vi "CRYTree Structure Update.vi"(8 "Is Refresh?":bool, 9 "Option":string, 10 "Add Items":T1(array[cluster]), 11 "StepsRef in":refnum<vi>) -> (0 "error out":errorcluster, 3 "StepsRefOut":refnum<vi>)   [LabVIEW 2013]
uses:
  <vilib>/Utility/miscctls.llb/LVNodeAndColumnTypeDef.ctl
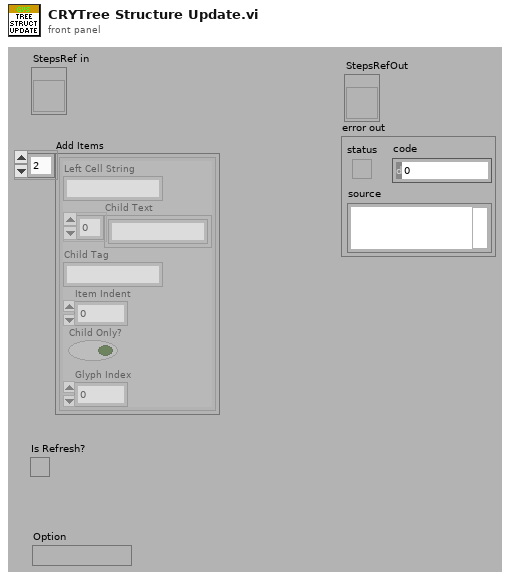
[diagram p1: front panel]
types:
  T1 = cluster{"Left Cell String":string, "Child Text":string[], "Child Tag":string, "Item Indent":i32, "Child Only?":bool, "Glyph Index":i32}[]
  T2 = typedef "LVNodeAndColumnTypeDef.ctl" = cluster{"Node":string, "Column":i32}
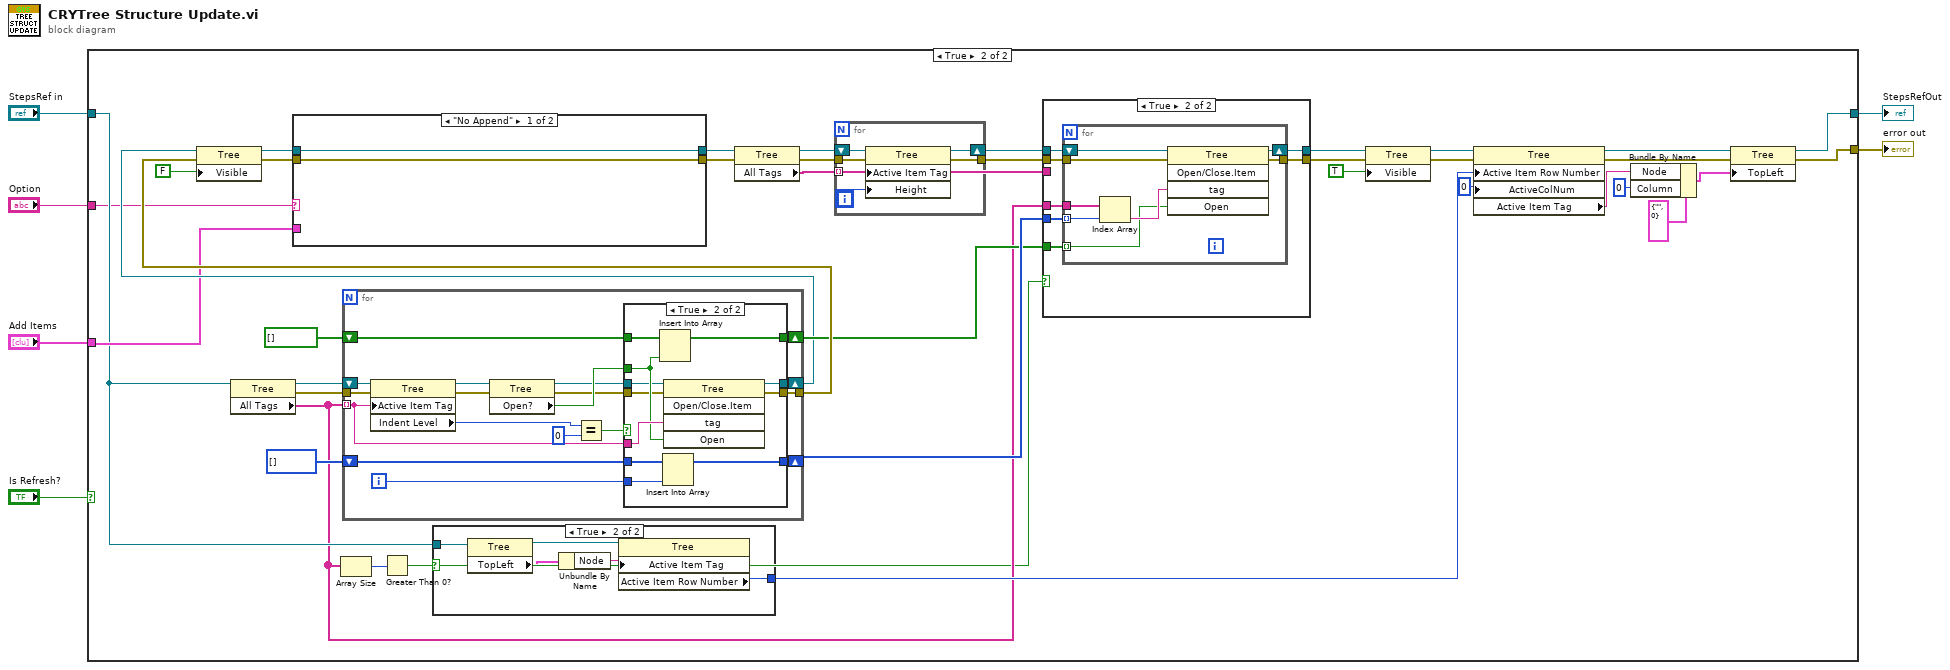
[diagram p0: block diagram]
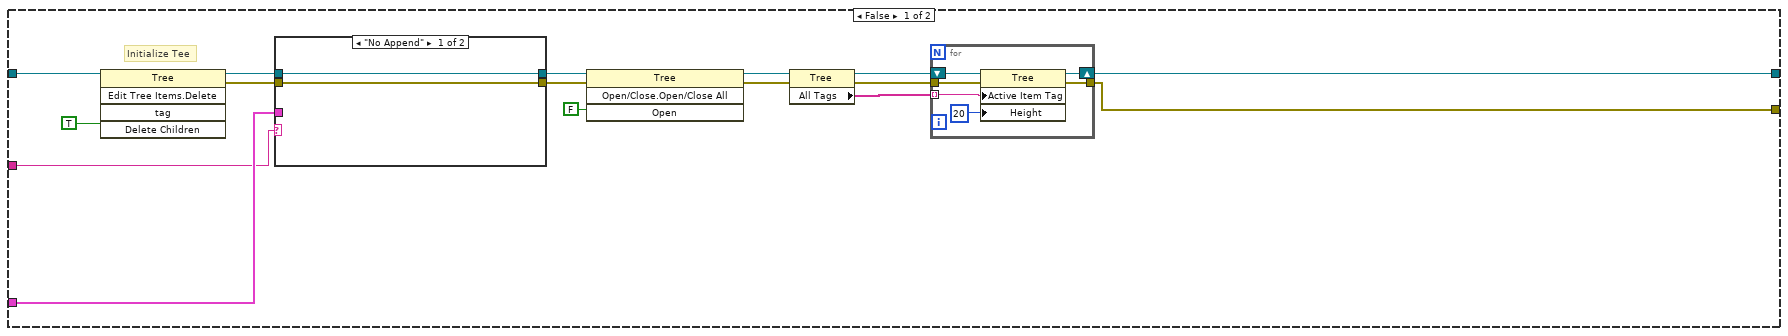
[diagram p2: hidden frame]
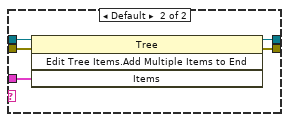
[diagram p3: hidden frame]
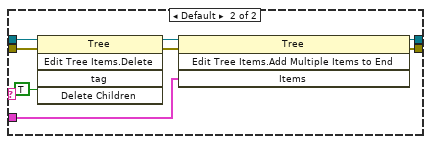
[diagram p4: hidden frame]
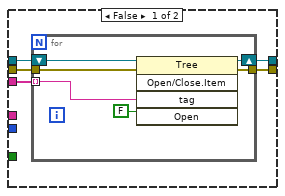
[diagram p5: hidden frame]
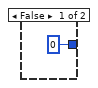
[diagram p6: hidden frame]
diagram:
  n1 = case shown="True" "Is Refresh?" {
    tunnel: [w22 w44] -> w6
    tunnel: "StepsRef in" -> [w21 w54]
    tunnel: [w20 w43] -> w4
    tunnel: "Add Items" -> [w8 w55]
    tunnel: "Option" -> [w7 w37]
    frame False {
      # "Initialize Tee"
      n2 = invoke class="Tree" method="Edit Tree Items.Delete"(reference=w21, "Delete Children"=TRUE ("Delete Children?")) -> (reference out=w14:refnum<vi>, error out=w12:errorcluster)  [unwired: 3 in, 3 out]
      n3 = case shown="\"No Append\"" w7 {
        tunnel: w14 -> [w24 w29]
        tunnel: [w24 w28] -> w13
        tunnel: w12 -> [w23 w27]
        tunnel: [w23 w26] -> w11
        tunnel: w8 -> [_ w25]
        frame "No Append" {
        }
        frame Default {
          n4 = invoke class="Tree" method="Edit Tree Items.Add Multiple Items to End"(reference=w29, error in=w27, "Items"=w25) -> (reference out=w28:refnum<vi>, error out=w26:errorcluster)  [unwired: 1 in, 2 out]
        }
      }
      n5 = invoke class="Tree" method="Open/Close.Open/Close All"(reference=w13, error in=w11, "Open"=FALSE ("Open?")) -> (reference out=w16:refnum<vi>, error out=w10:errorcluster)  [unwired: 1 in, 2 out]
      n6 = property class="Tree"(reference=w16, error in=w10) -> (reference out=w18:refnum<vi>, error out=w9:errorcluster, "All Tags"=w17:string[])
      n7 = for {
        tunnel: w17 -> [w32] mode=indexing
        shift-right: [w34] -> w22
        shift-left: w18 -> [w33]
        tunnel: w9 -> [w31]
        tunnel: [w30] -> w20
        n8 = property class="Tree"(reference=w33, error in=w31, "Active Item Tag"=w32, "Height"=20 ("Active Cell:Cell Size:Height")) -> (reference out=w34:refnum<vi>, error out=w30:errorcluster)
      }
    }
    frame True {
      n9 = property class="Tree"(reference=w54) -> (reference out=w58:refnum<vi>, error out=w69:errorcluster, "All Tags"=w41:string[])  [unwired: 1 in]
      n10 = Array Size(array=w41) -> (size(s)=w40:i32)
      n11 = for {
        tunnel: w41 -> [w129] mode=indexing
        shift-right: [w132] -> w65
        shift-left: bool[] [] ("Array") -> [w133]
        shift-right: [w130] -> w66
        shift-left: i32[] [] -> [w131]
        shift-right: [w127] -> w61
        shift-left: w58 -> [w139]
        tunnel: w69 -> [w126]
        tunnel: [w123] -> w70
        i -> [w135]
        n12 = property class="Tree"(reference=w139, error in=w126, "Active Item Tag"=w129) -> (reference out=w140:refnum<vi>, error out=w125:errorcluster, "Indent Level"=w138:i32)
        n13 = property class="Tree"(reference=w140, error in=w125) -> (reference out=w128:refnum<vi>, error out=w124:errorcluster, "Open?"=w134:bool)
        n14 = Equal?(x=w138, y=0) -> (x = y?=w136:bool)
        n15 = case shown="True" w136 {
          tunnel: w135 -> [_ w151]
          tunnel: w134 -> [_ w149]
          tunnel: w133 -> [w144 w155]
          tunnel: [w144 w154] -> w132
          tunnel: w131 -> [w143 w153]
          tunnel: [w143 w152] -> w130
          tunnel: w129 -> [_ w150]
          tunnel: w128 -> [w142 w148]
          tunnel: [w142 w147] -> w127
          tunnel: w124 -> [w141 w146]
          tunnel: [w141 w145] -> w123
          frame False {
          }
          frame True {
            n16 = Insert Into Array(array=w155, new element=w149) -> (w154:bool[])  [unwired: 1 in]
            n17 = Insert Into Array(array=w153, new element=w151) -> (w152:i32[])  [unwired: 1 in]
            n18 = invoke class="Tree" method="Open/Close.Item"(reference=w148, error in=w146, "tag"=w150, "Open"=w149) -> (reference out=w147:refnum<vi>, error out=w145:errorcluster)  [unwired: 1 in, 3 out]
          }
        }
      }
      n19 = property class="Tree"(reference=w61, error in=w70, "Visible"=FALSE) -> (reference out=w62:refnum<vi>, error out=w71:errorcluster)
      n20 = case shown="\"No Append\"" w37 {
        tunnel: [w75 w84] -> w72
        tunnel: w71 -> [w75 w82]
        tunnel: w62 -> [w76 w81]
        tunnel: [w76 w80] -> w60
        tunnel: w55 -> [_ w77]
        frame "No Append" {
        }
        frame Default {
          n21 = invoke class="Tree" method="Edit Tree Items.Delete"(reference=w81, error in=w82, "Delete Children"=TRUE ("Delete Children?")) -> (reference out=w79:refnum<vi>, error out=w83:errorcluster)  [unwired: 2 in, 3 out]
          n22 = invoke class="Tree" method="Edit Tree Items.Add Multiple Items to End"(reference=w79, error in=w83, "Items"=w77) -> (reference out=w80:refnum<vi>, error out=w84:errorcluster)  [unwired: 1 in, 2 out]
        }
      }
      n23 = Greater Than 0?(x=w40) -> (x > 0?=w39:bool)
      n24 = case shown="True" w39 {
        tunnel: w54 -> [_ w113]
        tunnel: [0 ("Active Item Row Number") w112] -> w45
        frame False {
        }
        frame True {
          n25 = property class="Tree"(reference=w113) -> (reference out=w115:refnum<vi>, "TopLeft"=w116:T2)  [unwired: 1 in, 1 out]
          n26 = Unbundle By Name(w116) -> ("Node"=w114:string)
          n27 = property on="Property Node" class="Tree"(reference=w115, "Active Item Tag"=w114) -> ("Active Item Row Number"=w112:i32)  [unwired: 1 in, 2 out]
        }
      }
      n28 = property class="Tree"(reference=w60, error in=w72) -> (reference out=w59:refnum<vi>, error out=w73:errorcluster, "All Tags"=w38:string[])
      n29 = for {
        tunnel: w38 -> [w119] mode=indexing
        shift-right: [w121] -> w67
        shift-left: w59 -> [w120]
        tunnel: w73 -> [w118]
        tunnel: [w117] -> w74
        n30 = property class="Tree"(reference=w120, error in=w118, "Active Item Tag"=w119, "Height"=20 ("Active Cell:Cell Size:Height")) -> (reference out=w121:refnum<vi>, error out=w117:errorcluster)
      }
      n31 = case shown="True" w39 {
        tunnel: [w86 w102] -> w36
        tunnel: w74 -> [w88 w101]
        tunnel: [w87 w100] -> w68
        tunnel: w67 -> [w89 w99]
        tunnel: w66 -> [_ w98]
        tunnel: w65 -> [_ w97]
        tunnel: w41 -> [_ w96]
        tunnel: w38 -> [w85 _]
        frame False {
          n32 = for {
            tunnel: w85 -> [w91] mode=indexing
            shift-right: [w95] -> w87
            shift-left: w89 -> [w94]
            tunnel: [w93] -> w86
            tunnel: w88 -> [w92]
            n33 = invoke class="Tree" method="Open/Close.Item"(reference=w94, error in=w92, "tag"=w91, "Open"=FALSE ("Open?")) -> (reference out=w95:refnum<vi>, error out=w93:errorcluster)  [unwired: 1 in, 3 out]
          }
        }
        frame True {
          n34 = for {
            tunnel: w97 -> [w107] mode=indexing
            tunnel: w98 -> [w109] mode=indexing
            tunnel: w96 -> [w110]
            shift-right: [w106] -> w100
            shift-left: w99 -> [w105]
            tunnel: [w104] -> w102
            tunnel: w101 -> [w103]
            n35 = Index Array(array=w110, index=w109) -> (element=w108:string)
            n36 = invoke class="Tree" method="Open/Close.Item"(reference=w105, error in=w103, "tag"=w108, "Open"=w107) -> (reference out=w106:refnum<vi>, error out=w104:errorcluster)  [unwired: 1 in, 3 out]
          }
        }
      }
      n37 = property class="Tree"(reference=w68, error in=w36, "Visible"=TRUE) -> (reference out=w47:refnum<vi>, error out=w46:errorcluster)
      n38 = property on="Property Node" class="Tree"(reference=w47, error in=w46, "Active Item Row Number"=w45, "ActiveColNum"=0 ("Active Cell:Active Column Number")) -> (reference out=w51:refnum<vi>, error out=w42:errorcluster, "Active Item Tag"=w52:string)
      n39 = Bundle By Name(cluster=T2 {"Node"="", "Column"=0} ("Top Left Visible Cell"), "Node"=w52, "Column"=0) -> (w50:T2)
      n40 = property class="Tree"(reference=w51, error in=w42, "TopLeft"=w50) -> (reference out=w44:refnum<vi>, error out=w43:errorcluster)
    }
  }
  "StepsRefOut" <- w6
  "error out" <- w4
